vi "2017visionprocessing.vi"(0 "Image In":T3, 1 "Red or Hue Range (Color Threshold 1)":cluster{"Lower value":i32, "Upper value":i32}={"Lower value"=239, "Upper value"=255}, 2 "Green or Sat Range (Color Threshold 1)":cluster{"Lower value":i32, "Upper value":i32}={"Lower value"=238, "Upper value"=255}, 3 "Blue or Luma or Val or Inten Range (Color Threshold 1)":cluster{"Lower value":i32, "Upper value":i32}={"Lower value"=241, "Upper value"=255}, 4 "Selection Values (Particle Filter 1)":T1(array[cluster])=[{"Measurement Parameter"=16, "Range Lower Value"=24.0, "Range Upper Value"=45.0, "Range"=FALSE, "Measurement Type"=FALSE}] {"Measurement Parameter" items=["Center of Mass X", "Center of Mass Y", "First Pixel X", "First Pixel Y", "Bounding Rect Left", "Bounding Rect Top", "Bounding Rect Right", "Bounding Rect Bottom", "Max Feret Diameter Start X", "Max Feret Diameter Start Y", "Max Feret Diameter End X", "Max Feret Diameter End Y", "Max Horiz. Segment Length Left", "Max Horiz. Segment Length Right", "Max Horiz. Segment Length Row", "-", "Bounding Rect Width", "Bounding Rect Height", "Bounding Rect Diagonal", "Perimeter", "Convex Hull Perimeter", "Holes' Perimeter", "Max Feret Diameter", "Equivalent Ellipse Major Axis", "Equivalent Ellipse Minor Axis", "Equivalent Ellipse Minor Axis (Feret)", "Equivalent Rect Long Side", "Equivalent Rect Short Side", "Equivalent Rect Diagonal", "Equivalent Rect Short Side (Feret)", "Average Horiz. Segment Length", "Average Vert. Segment Length", "Hydraulic Radius", "Waddel Disk Diameter", "-", "Area", "Holes' Area", "Particle & Holes' Area", "Convex Hull Area", "Image Area", "-", "Number of Holes", "Number of Horiz. Segments", "Number of Vert. Segments", "-", "Orientation", "Max Feret Diameter Orientation", "-", "% Area/Image Area", "% Area/(Particle & Holes' Area)", "Ratio of Equivalent Ellipse Axes", "Ratio of Equivalent Rect Sides", "-", "Elongation Factor", "Compactness Factor", "Heywood Circularity Factor", "Type Factor", "-", "Sum X", "Sum Y", "Sum XX", "Sum XY", "Sum YY", "Sum XXX", "Sum XXY", "Sum XYY", "Sum YYY", "-", "Moment of Inertia XX", "Moment of Inertia XY", "Moment of Inertia YY", "Moment of Inertia XXX", "Moment of Inertia XXY", "Moment of Inertia XYY", "Moment of Inertia YYY", "Norm. Moment of Inertia XX", "Norm. Moment of Inertia XY", "Norm. Moment of Inertia YY", "Norm. Moment of Inertia XXX", "Norm. Moment of Inertia XXY", "Norm. Moment of Inertia XYY", "Norm. Moment of Inertia YYY", "Hu Moment 1", "Hu Moment 2", "Hu Moment 3", "Hu Moment 4", "Hu Moment 5", "Hu Moment 6", "Hu Moment 7"]}, 5 "Selection Values (Particle Filter 2)":T1(array[cluster])=[{"Measurement Parameter"=17, "Range Lower Value"=22.0, "Range Upper Value"=640.0, "Range"=FALSE, "Measurement Type"=FALSE}] {"Measurement Parameter" items=["Center of Mass X", "Center of Mass Y", "First Pixel X", "First Pixel Y", "Bounding Rect Left", "Bounding Rect Top", "Bounding Rect Right", "Bounding Rect Bottom", "Max Feret Diameter Start X", "Max Feret Diameter Start Y", "Max Feret Diameter End X", "Max Feret Diameter End Y", "Max Horiz. Segment Length Left", "Max Horiz. Segment Length Right", "Max Horiz. Segment Length Row", "-", "Bounding Rect Width", "Bounding Rect Height", "Bounding Rect Diagonal", "Perimeter", "Convex Hull Perimeter", "Holes' Perimeter", "Max Feret Diameter", "Equivalent Ellipse Major Axis", "Equivalent Ellipse Minor Axis", "Equivalent Ellipse Minor Axis (Feret)", "Equivalent Rect Long Side", "Equivalent Rect Short Side", "Equivalent Rect Diagonal", "Equivalent Rect Short Side (Feret)", "Average Horiz. Segment Length", "Average Vert. Segment Length", "Hydraulic Radius", "Waddel Disk Diameter", "-", "Area", "Holes' Area", "Particle & Holes' Area", "Convex Hull Area", "Image Area", "-", "Number of Holes", "Number of Horiz. Segments", "Number of Vert. Segments", "-", "Orientation", "Max Feret Diameter Orientation", "-", "% Area/Image Area", "% Area/(Particle & Holes' Area)", "Ratio of Equivalent Ellipse Axes", "Ratio of Equivalent Rect Sides", "-", "Elongation Factor", "Compactness Factor", "Heywood Circularity Factor", "Type Factor", "-", "Sum X", "Sum Y", "Sum XX", "Sum XY", "Sum YY", "Sum XXX", "Sum XXY", "Sum XYY", "Sum YYY", "-", "Moment of Inertia XX", "Moment of Inertia XY", "Moment of Inertia YY", "Moment of Inertia XXX", "Moment of Inertia XXY", "Moment of Inertia XYY", "Moment of Inertia YYY", "Norm. Moment of Inertia XX", "Norm. Moment of Inertia XY", "Norm. Moment of Inertia YY", "Norm. Moment of Inertia XXX", "Norm. Moment of Inertia XXY", "Norm. Moment of Inertia XYY", "Norm. Moment of Inertia YYY", "Hu Moment 1", "Hu Moment 2", "Hu Moment 3", "Hu Moment 4", "Hu Moment 5", "Hu Moment 6", "Hu Moment 7"]}, 6 "Minimal Score (Shape Matching 1)":dbl=500.0, 7 "error in":errorcluster, 8 "Minimal Score (Shape Matching 2)":dbl=800.0) -> (20 "Image Out":T3, 21 "Number of Matches (Shape Matching 1)":i32, 22 "Shape Report (Shape Matching 1)":T2(array[cluster]) {"Score" format="%.2f"; "Centroid"."y" format="%.2f"; "Centroid"."x" format="%.2f"}, 23 "Shape Report (calibrated) (Shape Matching 1)":T2(array[cluster]) {"Score" format="%.2f"; "Centroid"."y" format="%.2f"; "Centroid"."x" format="%.2f"}, 24 "Number of Matches (Shape Matching 2)":i32, 25 "Shape Report (Shape Matching 2)":T2(array[cluster]) {"Score" format="%.2f"; "Centroid"."y" format="%.2f"; "Centroid"."x" format="%.2f"}, 26 "Shape Report (calibrated) (Shape Matching 2)":T2(array[cluster]) {"Score" format="%.2f"; "Centroid"."y" format="%.2f"; "Centroid"."x" format="%.2f"}, 27 "error out":errorcluster)   [LabVIEW 2016]
uses:
  <vilib>/vision/Image Controls.llb/IMAQ Image.ctl
  <vilib>/vision/NI_Vision_Development_Module.lvlib
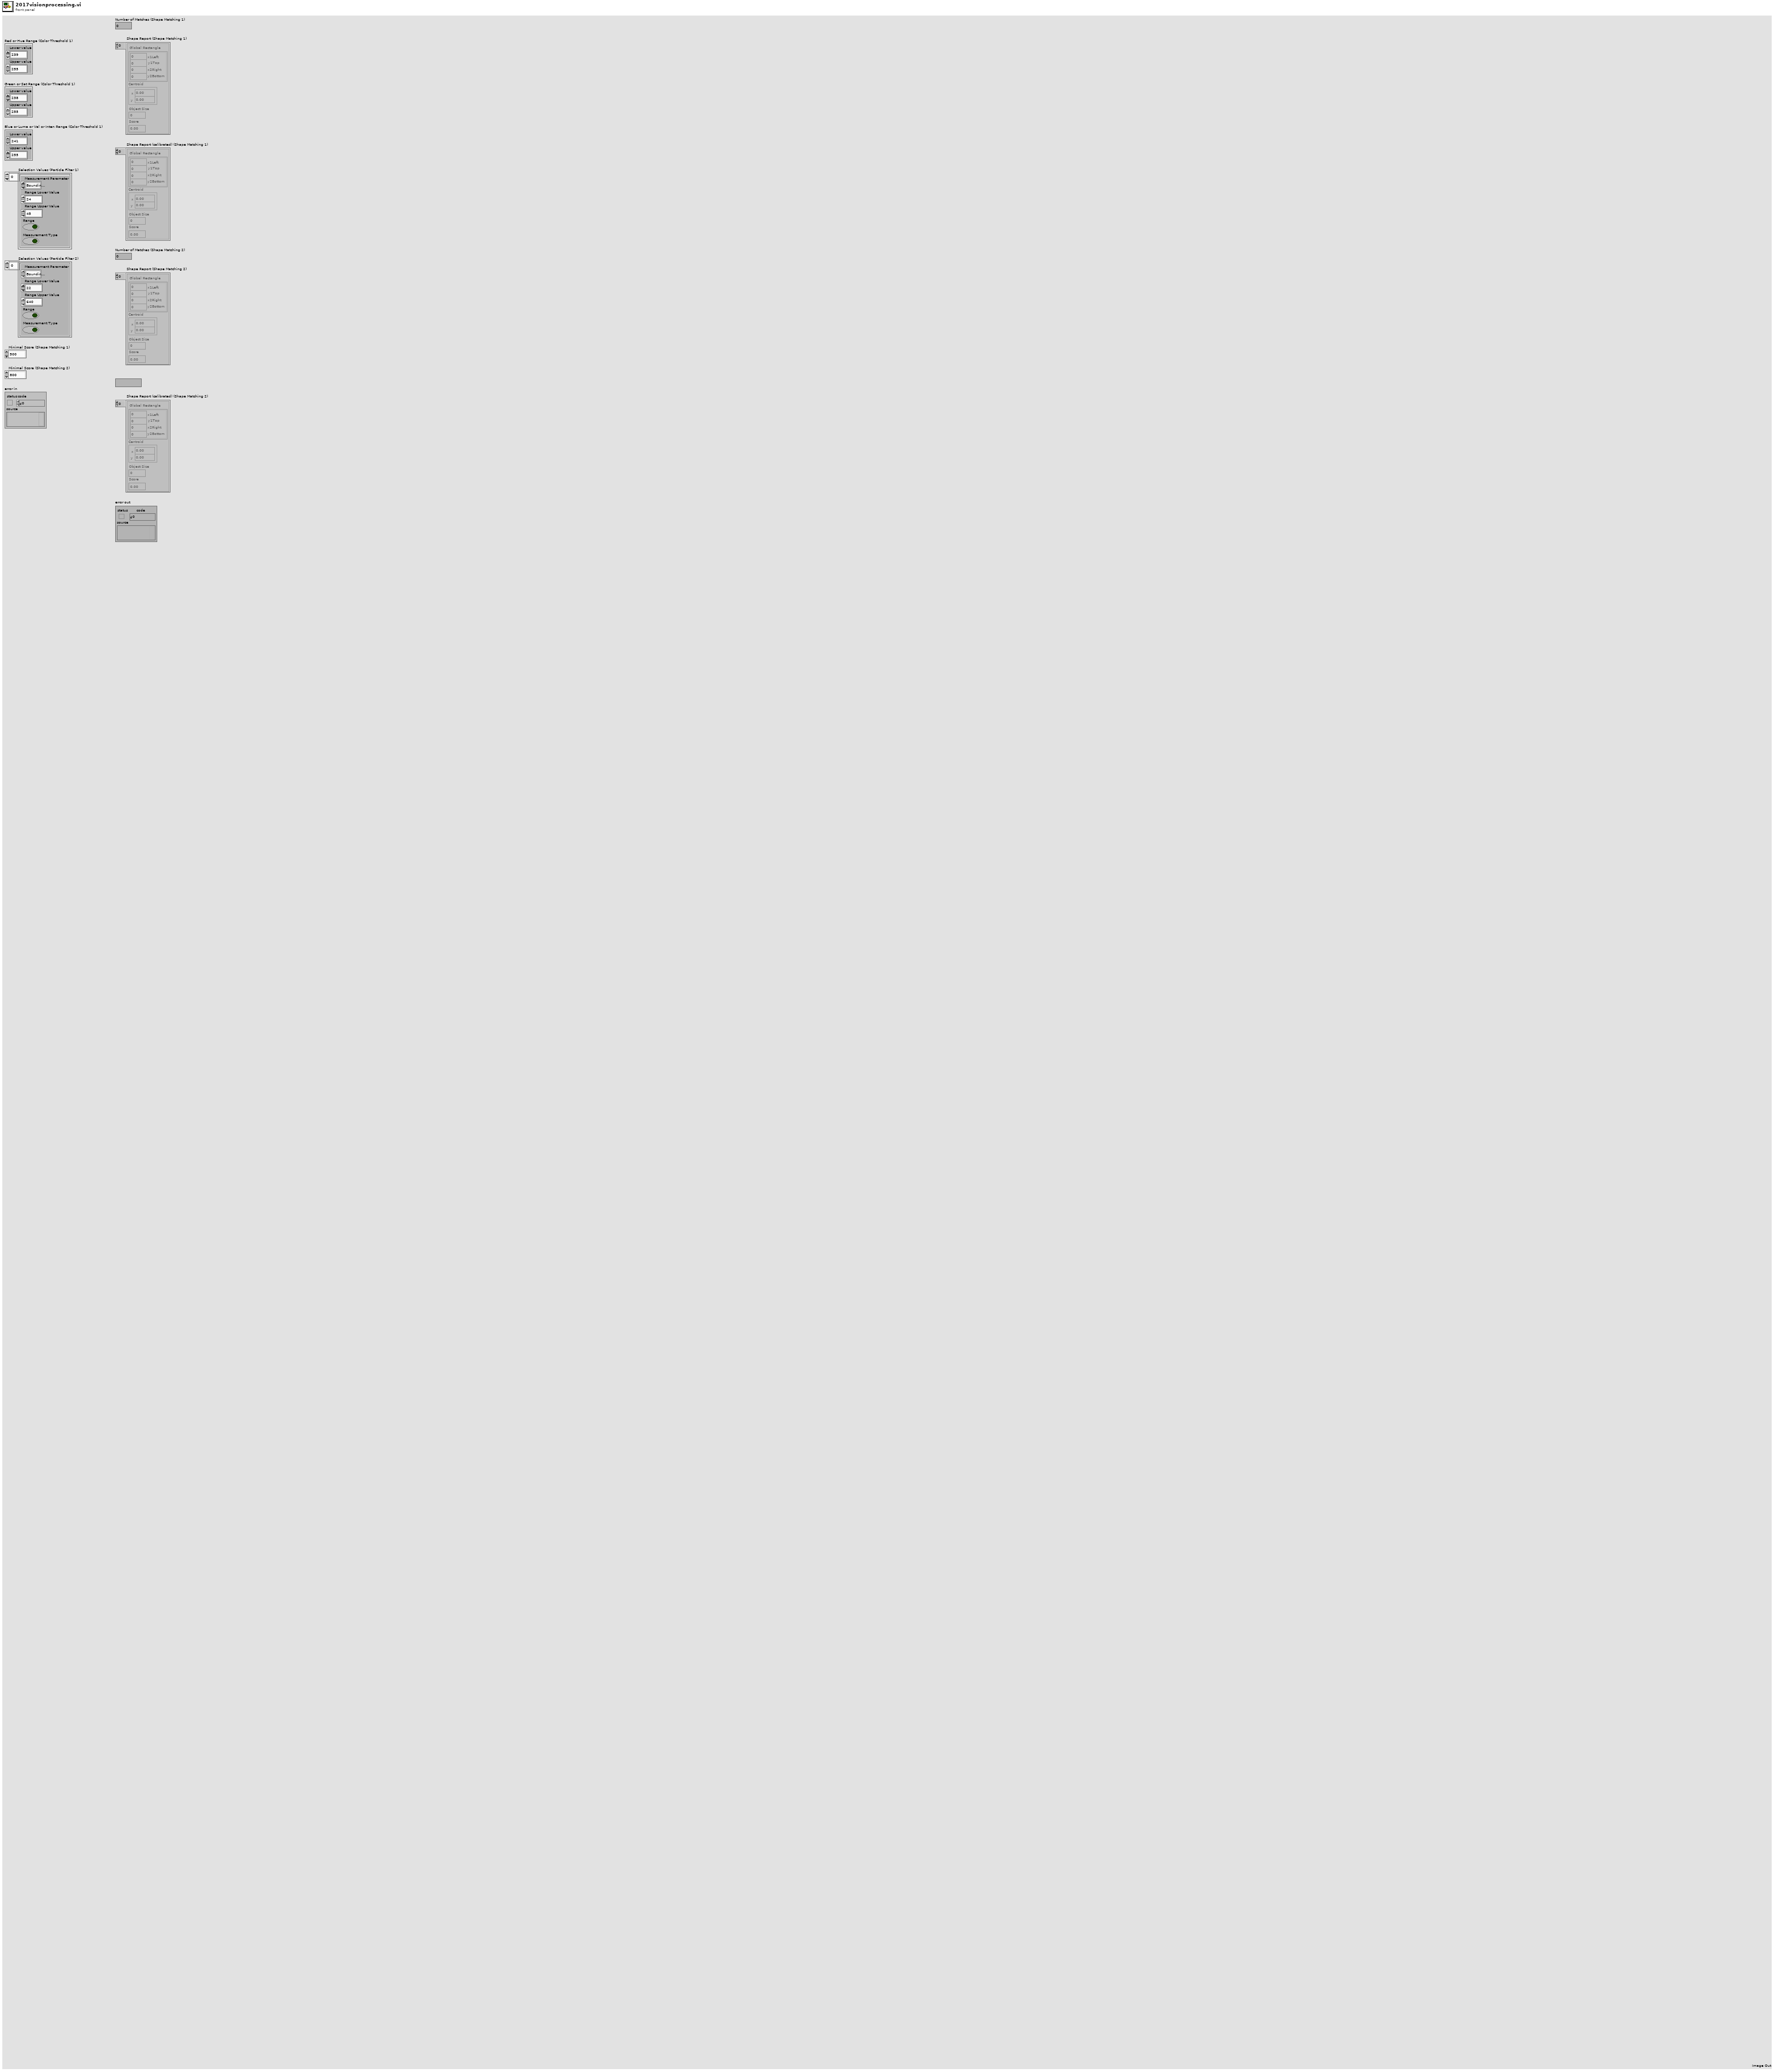
[diagram p1: front panel]
types:
  T1 = cluster{"Measurement Parameter":i32, "Range Lower Value":dbl, "Range Upper Value":dbl, "Range":bool, "Measurement Type":bool}[]
  T2 = cluster{"Global Rectangle":cluster{"x1Left":i32, "y1Top":i32, "x2Right":i32, "y2Bottom":i32}, "Centroid":cluster{"x":sgl, "y":sgl}, "Object Size":u32, "Score":dbl}[]
  T3 = typedef "IMAQ Image.ctl" = refnum<image>
  T4 = enum32{"AutoM", "Close", "Dilate", "Erode", "Gradient", "Gradient out", "Gradient in", "Hit miss", "Open", "PClose", "POpen", "Thick", "Thin"}
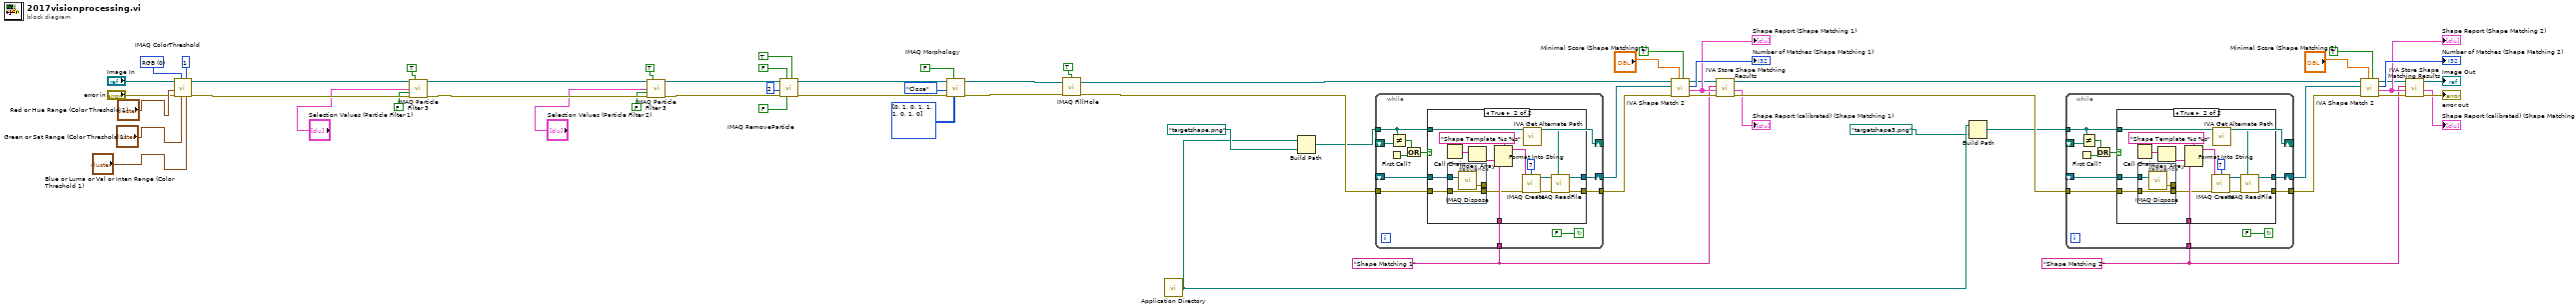
[diagram p0: block diagram]
diagram:
  w6 = "Shape Matching 2" ("Step Name")
  w19 = "Shape Matching 1" ("Step Name")
  w61 = u16 0 items=["RGB", "HSL", "HSV", "HSI"] ("Color Mode")
  n1 = call "IMAQ ColorThreshold"("Blue or Luma or Val or Inten Range"="Blue or Luma or Val or Inten Range (Color Threshold 1)", "Replace Value"=1, "Green or Sat Range"="Green or Sat Range (Color Threshold 1)", "Color Mode"=w61, "error in (no error)"="error in", "Red or Hue Range"="Red or Hue Range (Color Threshold 1)", "Image Src"="Image In") -> ("error out"=w55:errorcluster, "Image Dst Out"=w51:T3)  [unwired: 1 in, 2 out]
  n2 = call "IMAQ Particle Filter 3"("Image Src"=w51, "Connectivity 4/8 (8)"=TRUE, "Selection Values"="Selection Values (Particle Filter 1)", "Keep/Remove Particles (F)"=FALSE ("Keep/Remove Particles"), "error in (no error)"=w55) -> ("Image Dst Out"=w46:T3, "error out"=w52:errorcluster)  [unwired: 4 in, 5 out]
  n3 = call "IMAQ Particle Filter 3"("Image Src"=w46, "Connectivity 4/8 (8)"=TRUE, "Selection Values"="Selection Values (Particle Filter 2)", "Keep/Remove Particles (F)"=FALSE ("Keep/Remove Particles"), "error in (no error)"=w52) -> ("Image Dst Out"=w40:T3, "error out"=w47:errorcluster)  [unwired: 4 in, 5 out]
  n4 = call "IMAQ RemoveParticle"("Connectivity 4/8 (8)"=TRUE, "Low Pass/High Pass (Low)"=FALSE, "Square/Hexa (Square)"=FALSE, "error in (no error)"=w47, "Number of Erosion"=2, "Image Src"=w40) -> ("error out"=w39:errorcluster, "Image Dst Out"=w35:T3)  [unwired: 1 in, 3 out]
  n5 = call "IMAQ Morphology"("Structuring Element"=i32[][] [[0, 1, 0], [1, 1, 1], [0, 1, 0]], "Square/Hexa (Square)"=FALSE, "error in (no error)"=w39, "Operation"=T4."Close", "Image Src"=w35) -> ("error out"=w34:errorcluster, "Image Dst Out"=w32:T3)  [unwired: 2 in, 3 out]
  n6 = call "IMAQ FillHole"("error in (no error)"=w34, "Image Src"=w32, "Connectivity 4/8 (8)"=TRUE) -> ("error out"=w31:errorcluster, "Image Dst Out"=w27:T3)  [unwired: 1 in, 2 out]
  n7 = call <vilib>:"Application Directory.vi"() -> ("Application Directory"=w3:path)
  n8 = Build Path(base path=w3, name or relative path=path "targetshape.png" ("Template Path")) -> (appended path=w4:path)
  n9 = while {
    shift-right: [w73] -> w20
    shift-left: _ -> [w72]
    tunnel: [w70] -> w21
    tunnel: w31 -> [w69]
    tunnel: w4 -> [w67]
    tunnel: w19 -> [w68]
    shift-right: [w67] -> _
    shift-left: _ -> [w66]
    stop <- FALSE continue-if-true
    n10 = First Call?() -> (First Call?: T/F=w65:bool)
    n11 = Not Equal?(x=w67, y=w66) -> (x != y?=w64:bool)
    n12 = Or(x=w64, y=w65) -> (x .or. y?=w63:bool)
    n13 = case shown="True" w63 {
      tunnel: [w75 w87] -> w73
      tunnel: w72 -> [w75 w78]
      tunnel: [w74 w85] -> w70
      tunnel: w69 -> [w74 w77]
      tunnel: w67 -> [_ w80]
      tunnel: w68 -> [_ w81]
      frame False {
      }
      frame True {
        n14 = Call Chain() -> (call chain=w83:string[])
        n15 = stacked-sequence {
          tunnel: w78 -> [w93]
          tunnel: w77 -> [w92]
          tunnel: [w92] -> w76
          tunnel: [w91] -> _
          frame #0 {
            n16 = call "IMAQ Dispose"("Image"=w93) -> ("error out"=w91:errorcluster)  [unwired: 2 in, 3 out]
          }
        }
        n17 = Index Array(array=w83) -> (element=w82:string)  [unwired: 1 in]
        n18 = Format Into String(format string="Shape Template %s %s" ("Image Name"), w82, w81) -> (resulting string=w90:string)  [unwired: 2 in, 1 out]
        n19 = call "IMAQ Create"("Border Size"=7, "Image Name"=w90, "error in (no error)"=w76) -> ("New Image"=w88:T3, "error out"=w86:errorcluster)  [unwired: 1 in, 1 out]
        n20 = call <vilib>:"IVA Get Alternate Path.vi"("Path In"=w80) -> ("Path Out"=w79:path)  [unwired: 10 out]
        n21 = call "IMAQ ReadFile"("File Path"=w79, "error in (no error)"=w86, "Image"=w88) -> ("error out"=w85:errorcluster, "Image Out"=w87:T3)  [unwired: 2 in, 5 out]
      }
    }
  }
  n22 = call <vilib>:"IVA Shape Match 2.vi"("Scale Invariance"=TRUE, "Minimal Score"="Minimal Score (Shape Matching 1)", "error in (no error)"=w21, "Template"=w20, "Image Src"=w27) -> ("error out"=w26:errorcluster, "Shape Report"=w24:T2, "Number of Matches"=→"Number of Matches (Shape Matching 1)":i32, "Image Out"=w23:T3)  [unwired: 3 out]
  "Shape Report (Shape Matching 1)" <- w24
  n23 = call <vilib>:"IVA Store Shape Matching Results.vi"("error in (no error)"=w26, "Shape Report"=w24, "Step Name"=w19, "Image in"=w23) -> ("error out"=w25:errorcluster, "Shape Report (calibrated)"=→"Shape Report (calibrated) (Shape Matching 1)":T2, "Image dup"=w15:T3)  [unwired: 5 out]
  n24 = Build Path(base path=w3, name or relative path=path "targetshape3.png" ("Template Path")) -> (appended path=w1:path)
  n25 = while {
    shift-right: [w104] -> w7
    shift-left: _ -> [w103]
    tunnel: [w101] -> w8
    tunnel: w25 -> [w100]
    tunnel: w1 -> [w98]
    tunnel: w6 -> [w99]
    shift-right: [w98] -> _
    shift-left: _ -> [w97]
    stop <- FALSE continue-if-true
    n26 = First Call?() -> (First Call?: T/F=w96:bool)
    n27 = Not Equal?(x=w98, y=w97) -> (x != y?=w95:bool)
    n28 = Or(x=w95, y=w96) -> (x .or. y?=w94:bool)
    n29 = case shown="True" w94 {
      tunnel: [w106 w118] -> w104
      tunnel: w103 -> [w106 w109]
      tunnel: [w105 w116] -> w101
      tunnel: w100 -> [w105 w108]
      tunnel: w98 -> [_ w111]
      tunnel: w99 -> [_ w112]
      frame False {
      }
      frame True {
        n30 = Call Chain() -> (call chain=w114:string[])
        n31 = stacked-sequence {
          tunnel: w109 -> [w124]
          tunnel: w108 -> [w123]
          tunnel: [w123] -> w107
          tunnel: [w122] -> _
          frame #0 {
            n32 = call "IMAQ Dispose"("Image"=w124) -> ("error out"=w122:errorcluster)  [unwired: 2 in, 3 out]
          }
        }
        n33 = Index Array(array=w114) -> (element=w113:string)  [unwired: 1 in]
        n34 = Format Into String(format string="Shape Template %s %s" ("Image Name"), w113, w112) -> (resulting string=w121:string)  [unwired: 2 in, 1 out]
        n35 = call "IMAQ Create"("Border Size"=7, "Image Name"=w121, "error in (no error)"=w107) -> ("New Image"=w119:T3, "error out"=w117:errorcluster)  [unwired: 1 in, 1 out]
        n36 = call <vilib>:"IVA Get Alternate Path.vi"("Path In"=w111) -> ("Path Out"=w110:path)  [unwired: 10 out]
        n37 = call "IMAQ ReadFile"("File Path"=w110, "error in (no error)"=w117, "Image"=w119) -> ("error out"=w116:errorcluster, "Image Out"=w118:T3)  [unwired: 2 in, 5 out]
      }
    }
  }
  n38 = call <vilib>:"IVA Shape Match 2.vi"("Scale Invariance"=TRUE, "Minimal Score"="Minimal Score (Shape Matching 2)", "error in (no error)"=w8, "Template"=w7, "Image Src"=w15) -> ("error out"=w14:errorcluster, "Shape Report"=w12:T2, "Number of Matches"=→"Number of Matches (Shape Matching 2)":i32, "Image Out"=w11:T3)  [unwired: 3 out]
  "Shape Report (Shape Matching 2)" <- w12
  n39 = call <vilib>:"IVA Store Shape Matching Results.vi"("error in (no error)"=w14, "Shape Report"=w12, "Step Name"=w6, "Image in"=w11) -> ("error out"=→"error out":errorcluster, "Shape Report (calibrated)"=→"Shape Report (calibrated) (Shape Matching 2)":T2, "Image dup"=→"Image Out":T3)  [unwired: 5 out]
